vi "read-sort-data-v2.vi"(7 "all-data in":T1 {"dP3"."Temp (degC)" format="%.2f"; "dP3"."dP (mBar)" format="%.2f"; "dP2"."Temp (degC)" format="%.2f"; "dP2"."dP (mBar)" format="%.2f"; "dP1"."Temp (degC)" format="%.2f"; "dP1"."dP (mBar)" format="%.2f"; "CD4"."CO2 (ppm)" format="%.2f"; "CD3"."CO2 (ppm)" format="%.2f"; "RHT4"."Humidity (%)" format="%.2f"; "RHT4"."Temp (degC)" format="%.2f"; "RHT5"."Humidity (%)" format="%.2f"; "RHT5"."Temp (degC)" format="%.2f"; "CD2"."Humidity (%)" format="%.2f"; "CD2"."Temp (degC)" format="%.2f"; "CD2"."CO2 (ppm)" format="%.2f"; "RHT3"."Humidity (%)" format="%.2f"; "RHT3"."Temp (degC)" format="%.2f"; "CD6"."CO2 (ppm)" format="%.2f"; "RHT6"."Humidity (%)" format="%.2f"; "RHT6"."Temp (degC)" format="%.2f"; "CD5"."CO2 (ppm)" format="%.2f"; "CD1"."Humidity (%)" format="%.2f"; "CD1"."Temp (degC)" format="%.2f"; "CD1"."CO2 (ppm)" format="%.2f"}, 8 "error in (no error)":errorcluster, 11 "VISA Refnum in":refnum<visa-resource-name>) -> (0 "error out":errorcluster, 1 "timestamp":i32, 2 "all-data out":T1 {"dP3"."Temp (degC)" format="%.2f"; "dP3"."dP (mBar)" format="%.2f"; "dP2"."Temp (degC)" format="%.2f"; "dP2"."dP (mBar)" format="%.2f"; "dP1"."Temp (degC)" format="%.2f"; "dP1"."dP (mBar)" format="%.2f"; "CD4"."CO2 (ppm)" format="%.2f"; "CD3"."CO2 (ppm)" format="%.2f"; "RHT4"."Humidity (%)" format="%.2f"; "RHT4"."Temp (degC)" format="%.2f"; "RHT5"."Humidity (%)" format="%.2f"; "RHT5"."Temp (degC)" format="%.2f"; "CD2"."Humidity (%)" format="%.2f"; "CD2"."Temp (degC)" format="%.2f"; "CD2"."CO2 (ppm)" format="%.2f"; "RHT3"."Humidity (%)" format="%.2f"; "RHT3"."Temp (degC)" format="%.2f"; "CD6"."CO2 (ppm)" format="%.2f"; "RHT6"."Humidity (%)" format="%.2f"; "RHT6"."Temp (degC)" format="%.2f"; "CD5"."CO2 (ppm)" format="%.2f"; "CD1"."Humidity (%)" format="%.2f"; "CD1"."Temp (degC)" format="%.2f"; "CD1"."CO2 (ppm)" format="%.2f"}, 3 "VISA Refnum out":refnum<visa-resource-name>, 4 "read buffer":string)   [LabVIEW 2021]
uses:
  all-sensor-data.ctl
  SCD41.ctl
  STC31.ctl
  SHT41.ctl
  SDP810.ctl
panel:
  out "read buffer out":string
  out "Bytes Returned":u32
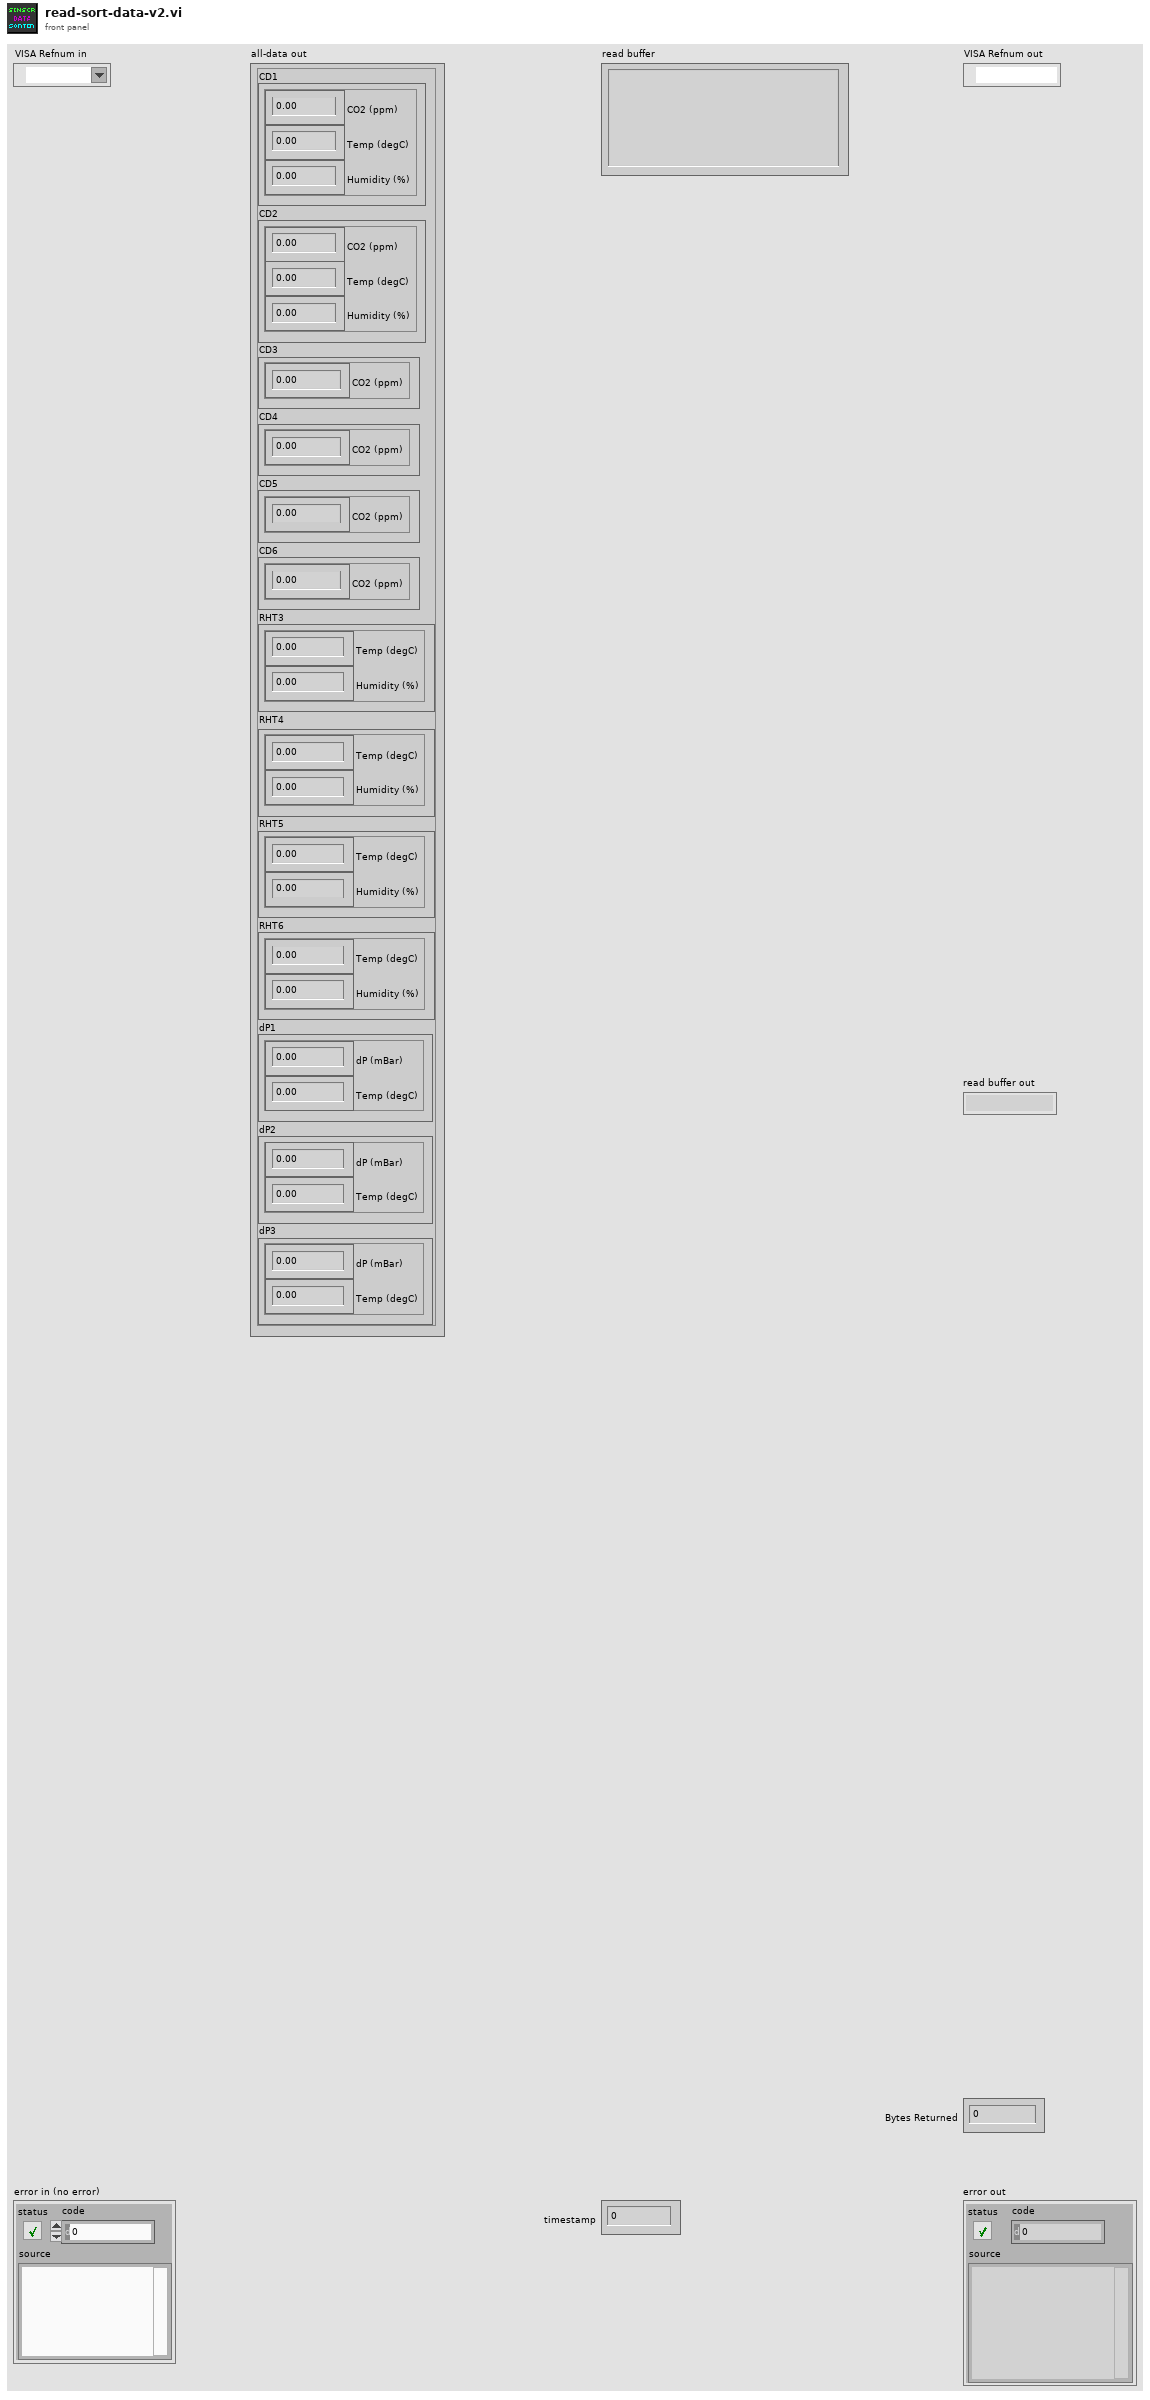
[diagram p1: front panel]
types:
  T1 = typedef "all-sensor-data.ctl" = cluster{"CD1":T2, "CD2":T2, "CD3":T3, "CD4":T3, "CD5":T3, "CD6":T3, "RHT3":T4, "RHT4":T4, "RHT5":T4, "RHT6":T4, "dP1":T5, "dP2":T5, "dP3":T5}
  T2 = typedef "SCD41.ctl" = cluster{"CO2 (ppm)":dbl, "Temp (degC)":dbl, "Humidity (%)":dbl}
  T3 = typedef "STC31.ctl" = cluster{"CO2 (ppm)":dbl}
  T4 = typedef "SHT41.ctl" = cluster{"Temp (degC)":dbl, "Humidity (%)":dbl}
  T5 = typedef "SDP810.ctl" = cluster{"dP (mBar)":dbl, "Temp (degC)":dbl}
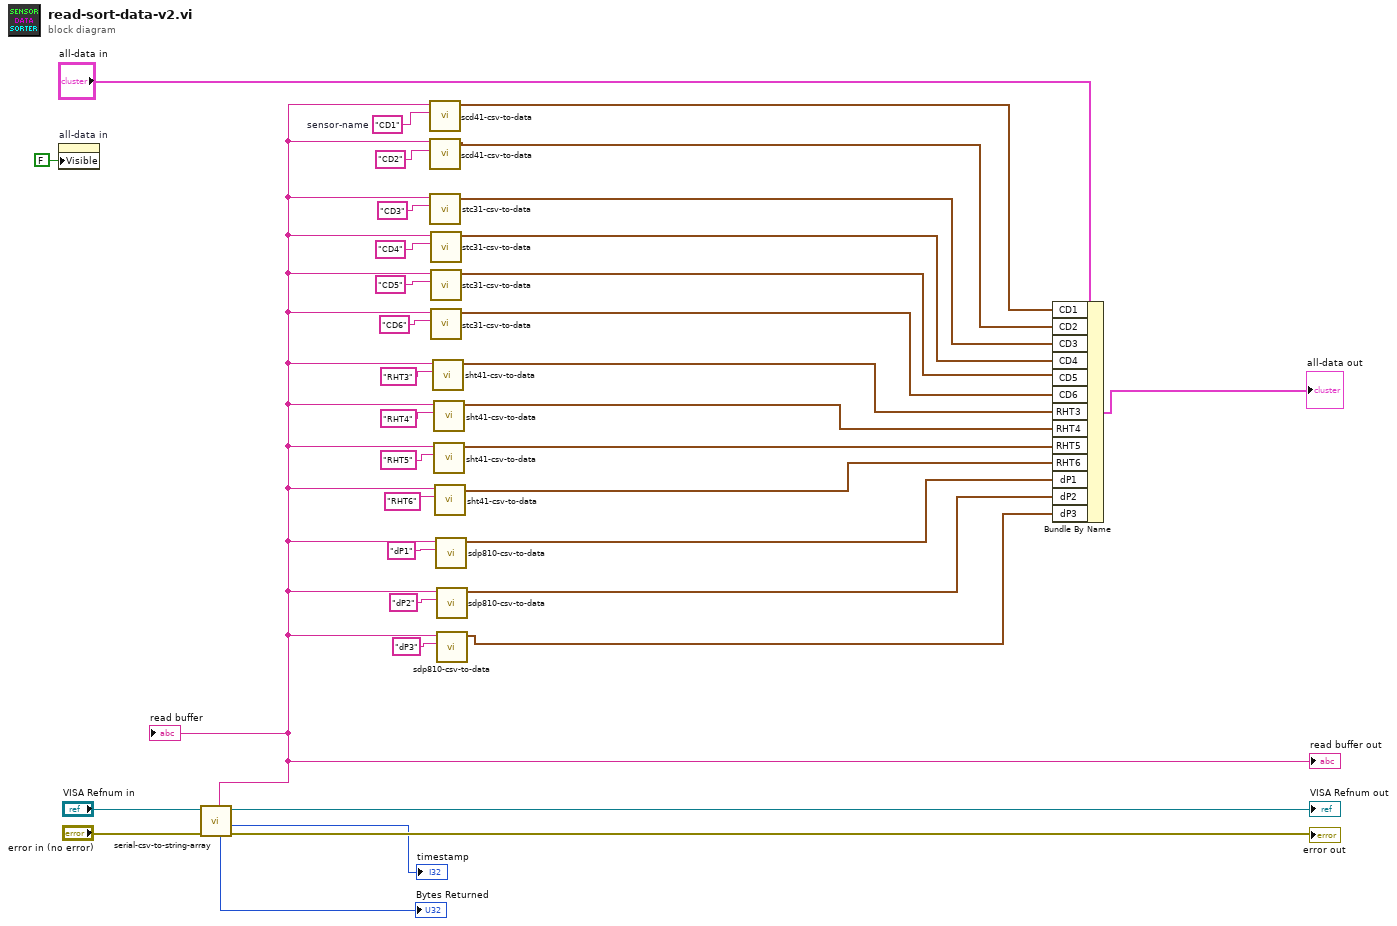
[diagram p0: block diagram]
diagram:
  w27 = "CD1"  # sensor-name
  n1 = property on="all-data in" class="Clust (strict)"("Visible"=FALSE) -> ()  [unwired: 2 in, 2 out]
  n2 = call "serial-csv-to-string-array.vi"("error in (no error)"="error in (no error)", "VISA Refnum in"="VISA Refnum in") -> ("error out"=→"error out":errorcluster, "timestamp"=→"timestamp":i32, "VISA Refnum out"=→"VISA Refnum out":refnum<visa-resource-name>, "Bytes Returned"=→"Bytes Returned":u32, "read buffer"=w5:string)  [unwired: 4 in, 1 out]
  "read buffer" <- w5
  "read buffer out" <- w5
  n3 = call "scd41-csv-to-data.vi"("sensor-name"=w27, "sensor-csv-input"=w5) -> ("SCD typedef"=w1:T2)  [unwired: 6 in, 3 out]
  n4 = call "scd41-csv-to-data.vi"("sensor-name"="CD2", "sensor-csv-input"=w5) -> ("SCD typedef"=w25:T2)  [unwired: 6 in, 3 out]
  n5 = call "stc31-csv-to-data.vi"("sensor-name"="CD3", "sensor-csv-input"=w5) -> ("STC31: data output"=w24:T3)  [unwired: 7 in, 2 out]
  n6 = call "stc31-csv-to-data.vi"("sensor-name"="CD4", "sensor-csv-input"=w5) -> ("STC31: data output"=w23:T3)  [unwired: 7 in, 2 out]
  n7 = call "stc31-csv-to-data.vi"("sensor-name"="CD5", "sensor-csv-input"=w5) -> ("STC31: data output"=w22:T3)  [unwired: 7 in, 2 out]
  n8 = call "stc31-csv-to-data.vi"("sensor-name"="CD6", "sensor-csv-input"=w5) -> ("STC31: data output"=w21:T3)  [unwired: 7 in, 2 out]
  n9 = call "sht41-csv-to-data.vi"("sensor-name"="RHT3" ("sensor-csv-input"), "sensor-csv-input"=w5) -> ("SHT41: data output"=w16:T4)  [unwired: 7 in, 2 out]
  n10 = call "sht41-csv-to-data.vi"("sensor-name"="RHT4" ("sensor-csv-input"), "sensor-csv-input"=w5) -> ("SHT41: data output"=w15:T4)  [unwired: 7 in, 2 out]
  n11 = call "sht41-csv-to-data.vi"("sensor-name"="RHT5" ("sensor-csv-input"), "sensor-csv-input"=w5) -> ("SHT41: data output"=w14:T4)  [unwired: 7 in, 2 out]
  n12 = call "sht41-csv-to-data.vi"("sensor-name"="RHT6" ("sensor-csv-input"), "sensor-csv-input"=w5) -> ("SHT41: data output"=w13:T4)  [unwired: 7 in, 2 out]
  n13 = call "sdp810-csv-to-data.vi"("sensor-name"="dP1", "sensor-csv-input"=w5) -> ("SDP810: data output"=w6:T4)  [unwired: 7 in, 2 out]
  n14 = call "sdp810-csv-to-data.vi"("sensor-name"="dP2", "sensor-csv-input"=w5) -> ("SDP810: data output"=w7:T4)  [unwired: 7 in, 2 out]
  n15 = call "sdp810-csv-to-data.vi"("sensor-name"="dP3", "sensor-csv-input"=w5) -> ("SDP810: data output"=w8:T4)  [unwired: 7 in, 2 out]
  n16 = Bundle By Name(cluster="all-data in", "CD1"=w1, "CD2"=w25, "CD3"=w24, "CD4"=w23, "CD5"=w22, "CD6"=w21, "RHT3"=w16, "RHT4"=w15, "RHT5"=w14, "RHT6"=w13, "dP1"=w6, "dP2"=w7, "dP3"=w8) -> (→"all-data out":T1)
